vi "niDTS BT EDR Tx Test Get Default Limits.vi"(0 "Dummy Test Handle In":T6, 11 "error in (no error)":errorcluster) -> (4 "Dummy Test Handle Out":T6, 6 "USL":T1, 8 "LSL":T1, 15 "error out":errorcluster)   [LabVIEW 2014, in "niDTS BT.lvlib"]
uses:
  niDTS BT.lvlib
  Tx Test/Includes/niDTS BT Tx Test INC Handle.ctl
  Tx Test/Objects/BASE_class/niDTS BT Tx Test.lvclass
  Includes/niDTS BT EDR Tx Test INC Results.ctl
  Tx Test/Includes/niDTS BT Tx Test INC IBE Results.ctl
  Tx Test/Includes/niDTS BT Tx Test INC DEVM Results.ctl
  Tx Test/Includes/niDTS BT Tx Test INC CF Stability Results.ctl
  Tx Test/Includes/niDTS BT Tx Test INC TXP Results.ctl
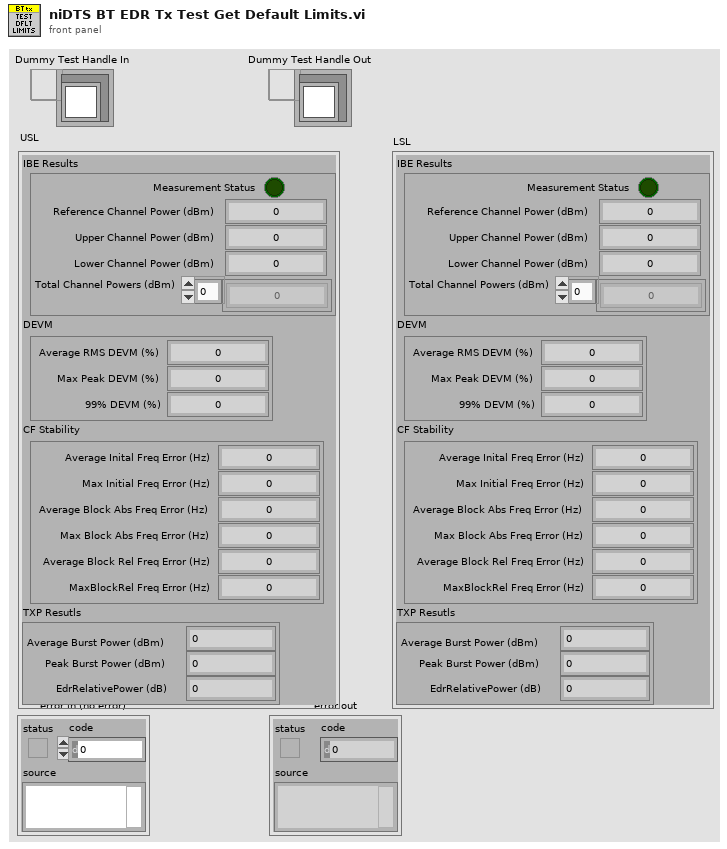
[diagram p1: front panel]
types:
  T1 = typedef "niDTS BT.lvlib/niDTS BT EDR Tx Test INC Results.ctl" = cluster{"IBE Results":T2, "DEVM":T3, "CF Stability":T4, "TXP Resutls":T5}
  T2 = typedef "niDTS BT.lvlib/niDTS BT Tx Test INC IBE Results.ctl" = cluster{"Measurement Status":bool, "Reference Channel Power (dBm)":dbl, "Upper Channel Power (dBm)":dbl, "Lower Channel Power (dBm)":dbl, "Total Channel Powers (dBm)":dbl[]}
  T3 = typedef "niDTS BT.lvlib/niDTS BT Tx Test INC DEVM Results.ctl" = cluster{"Average RMS DEVM (%)":dbl, "Max Peak DEVM (%)":dbl, "99% DEVM (%)":dbl}
  T4 = typedef "niDTS BT.lvlib/niDTS BT Tx Test INC CF Stability Results.ctl" = cluster{"Average Inital Freq Error (Hz)":dbl, "Max Initial Freq Error (Hz)":dbl, "Average Block Abs Freq Error (Hz)":dbl, "Max Block Abs Freq Error (Hz)":dbl, "Average Block Rel Freq Error (Hz)":dbl, "MaxBlockRel Freq Error (Hz)":dbl}
  T5 = typedef "niDTS BT.lvlib/niDTS BT Tx Test INC TXP Results.ctl" = cluster{"Average Burst Power (dBm)":dbl, "Peak Burst Power (dBm)":dbl, "EdrRelativePower (dB)":dbl}
  T6 = typedef "niDTS BT.lvlib/niDTS BT Tx Test INC Handle.ctl" = refnum<data-value>
  T7 = typedef "niDTS BT.lvlib/niDTS BT Tx Test INC Results.ctl" = cluster{"IBE Results":T2, "OBW Resutls":T8, "TXP Resutls":T5, "DEVM":T3, "CF Stability":T4, "CFO":T9, "DF1/DF2":T10}
  T8 = typedef "niDTS BT.lvlib/niDTS BT Tx Test INC OBW Results.ctl" = cluster{"OBW (Hz)":dbl, "Start Frequency (Hz)":dbl, "Stop Frequency (Hz)":dbl}
  T9 = typedef "niDTS BT.lvlib/niDTS BT Tx Test INC CFO Resutls.ctl" = cluster{"Max ICFT (Hz)":dbl, "Max Carrier Drift (Hz)":dbl, "Max Carrier Drift/50us (Hz)":dbl, "LE MaxPayloadBlockFreqOffset (Hz)":dbl, "LE MaxCarrierDrift/55us (Hz)":dbl}
  T10 = typedef "niDTS BT.lvlib/niDTS BT Tx Test INC Character Results.ctl" = cluster{"Average df1Avg (Hz)":dbl, "Max df1Max (Hz)":dbl, "Min df1Max (Hz)":dbl, "Measurement Status df1":bool, "Average  df2Avg/Average df1Avg":dbl, "Average df2Avg (Hz)":dbl, "Max df2Max (Hz)":dbl, "Min df2Max (Hz)":dbl, "Measurement Status df2":bool}
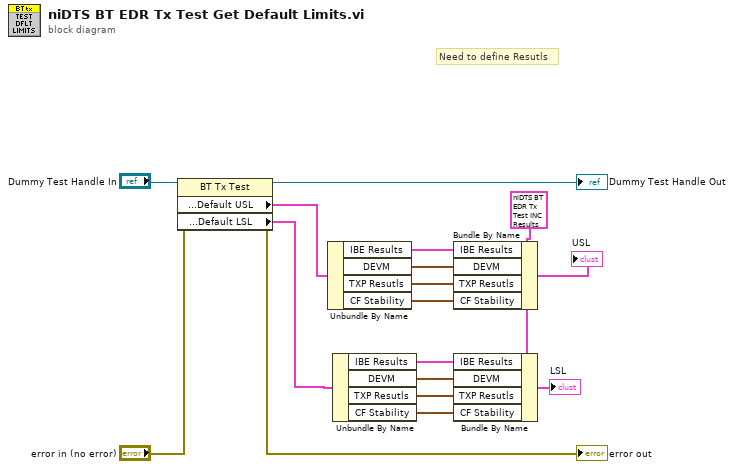
[diagram p0: block diagram]
diagram:
  w5 = T1 {"IBE Results"={"Measurement Status"=FALSE, "Reference Channel Power (dBm)"=0.0, "Upper Channel Power (dBm)"=0.0, "Lower Channel Power (dBm)"=0.0, "Total Channel Powers (dBm)"=[]}, "DEVM"={"Average RMS DEVM (%)"=0.0, "Max Peak DEVM (%)"=0.0, "99% DEVM (%)"=0.0}, "CF Stability"={"Average Inital Freq Error (Hz)"=0.0, "Max Initial Freq Error (Hz)"=0.0, "Average Block Abs Freq Error (Hz)"=0.0, "Max Block Abs Freq Error (Hz)"=0.0, "Average Block Rel Freq Error (Hz)"=0.0, "MaxBlockRel Freq Error (Hz)"=0.0}, "TXP Resutls"={"Average Burst Power (dBm)"=0.0, "Peak Burst Power (dBm)"=0.0, "EdrRelativePower (dB)"=0.0}} ("USL 2")
  # "Need to define Resutls"
  n1 = property class="BT Tx Test"(reference="Dummy Test Handle In", error in="error in (no error)") -> (reference out=→"Dummy Test Handle Out":T6, error out=→"error out":errorcluster, "Properties:Default Limits:Default USL"=w15:T7, "Properties:Default Limits:Default LSL"=w6:T7)
  n2 = Unbundle By Name(w15) -> ("IBE Results"=w12:T2, "DEVM"=w11:T3, "TXP Resutls"=w10:T5, "CF Stability"=w2:T4)
  n3 = Unbundle By Name(w6) -> ("IBE Results"=w9:T2, "DEVM"=w8:T3, "TXP Resutls"=w7:T5, "CF Stability"=w1:T4)
  n4 = Bundle By Name(cluster=w5, "IBE Results"=w12, "DEVM"=w11, "TXP Resutls"=w10, "CF Stability"=w2) -> (→"USL":T1)
  n5 = Bundle By Name(cluster=w5, "IBE Results"=w9, "DEVM"=w8, "TXP Resutls"=w7, "CF Stability"=w1) -> (→"LSL":T1)
